vi "IncrementArray.vi"(1 "Increment":dbl, 2 "End":dbl, 3 "Start":dbl) -> (0 "Array":dbl[](array[numeric]))   [LabVIEW 2023]
panel:
  out "size(s)":i32
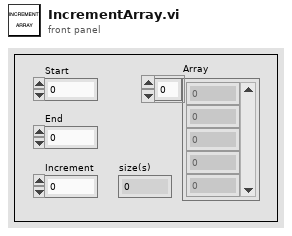
[diagram p1: front panel]
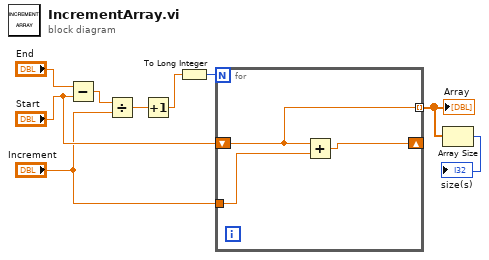
[diagram p0: block diagram]
diagram:
  n1 = Subtract(x="End", y="Start") -> (x-y=w8:dbl)
  n2 = Divide(x=w8, y="Increment") -> (x/y=w7:dbl)
  n3 = Increment(x=w7) -> (x+1=w4:dbl)
  n4 = To Long Integer(number=w4) -> (32bit integer=w3:i32)
  n5 = for {
    N: w3 -> [_]
    shift-right: [w11] -> _
    shift-left: "Start" -> [w10]
    tunnel: "Increment" -> [w12]
    tunnel: [w10] -> w2 mode=indexing
    n6 = Add(x=w10, y=w12) -> (x+y=w11:dbl)
  }
  "Array" <- w2
  n7 = Array Size(array=w2) -> (size(s)=→"size(s)":i32)
